vi "Union_TAGs_RFIDs.vi"(1 "TAGs LR6":string[](array[string]), 2 "TAGs HEX":string[](array[string])) -> (0 "TAGs":string[](array[string]))   [LabVIEW 2015]
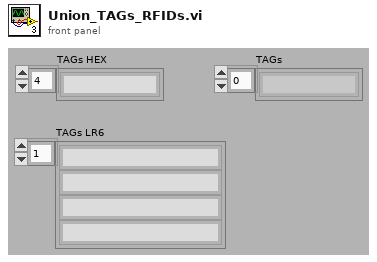
[diagram p1: front panel]
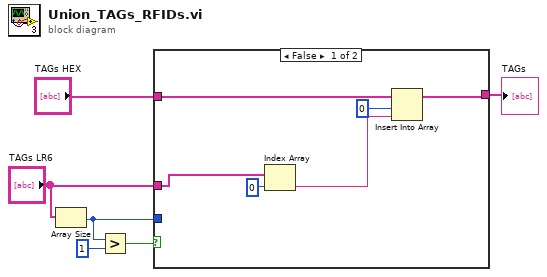
[diagram p0: block diagram]
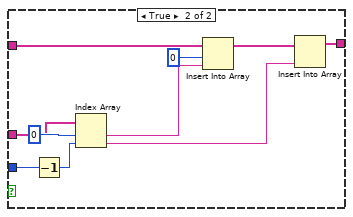
[diagram p2: hidden frame]
diagram:
  n1 = Array Size(array="TAGs LR6") -> (size(s)=w3:i32)
  n2 = Greater?(x=w3, y=1) -> (0:w2:bool)
  n3 = case shown="False" w2 {
    tunnel: w3 -> [_ w21]
    tunnel: "TAGs LR6" -> [w8 w19]
    tunnel: "TAGs HEX" -> [w9 w18]
    tunnel: [w7 w13] -> w4
    frame False {
      n4 = Index Array(array=w8, index=0) -> (element=w11:string)
      n5 = Insert Into Array(array=w9, index=0, new element=w11) -> (w7:string[])
    }
    frame True {
      n6 = Decrement(x=w21) -> (x-1=w20:i32)
      n7 = Index Array(array=w19, index #1=0 ("index"), index #2=w20) -> (element #1=w17:string, element #2=w14:string)
      n8 = Insert Into Array(array=w18, index=0, new element=w17) -> (w15:string[])
      n9 = Insert Into Array(array=w15, new element=w14) -> (w13:string[])  [unwired: 1 in]
    }
  }
  "TAGs" <- w4
